vi "Bind Terminal Enabled State.vi"(4 "FALSE State (Disabled and Grayed Out)":T1(ring), 6 "TRUE State (Enabled)":T1(ring), 7 "Initial State (T)":bool=TRUE, 8 "error in (no error)":errorcluster, 9 "Datum Name (\"\"=Use Control Label)":string, 10 "Ctl Refnum":refnum<vi>, 11 "IViewable in":refnum<class "IViewable.lvclass">) -> (0 "error out":errorcluster, 3 "IViewable out":refnum<class "IViewable.lvclass">)   [LabVIEW 2015, in "IViewable.lvlib" / "IViewable.lvclass"]
doc: "Bind the enabled state of a control terminal (control or indicator) to a published Boolean or Numeric datum. Specify the logical relationship between datum vale and terminal state by wiring the optional input terminals.\n\nDefault for Boolean:\nPublished TRUE = Enabled\nPublished FALSE = Disabled and Grayed Out\n\nDefault for Numeric:\nPublised value greater than 0 = Enabled\nPublished value NOT greater than 0 = Disabled and Grayed Out"
uses:
  IViewable.lvclass
  <vilib>/ActorFramework/Actor/Actor.lvclass/Actor.ctl
  <vilib>/ActorFramework/Message Enqueuer/Message Enqueuer.lvclass/Message Enqueuer.ctl
  SubscriptionPolicy/ValueChangeSubscription/ValueChangeSubscription.lvclass/ValueChangeSubscription.ctl
  IMediator/SubscriptionRequest/SubscriptionRequest.lvclass/SubscriptionRequest.ctl
  IObserver/IObserver Messages/Subscribe Msg/Subscribe Msg.lvclass/Subscribe Msg.ctl
  <vilib>/ActorFramework/Message Enqueuer/Init from Existing Queue.vi
  <vilib>/ActorFramework/Message Enqueuer/Enqueue.vi
  <vilib>/ActorFramework/Message Priority Queue/Priority Enqueue.vi
  SubscriptionPolicy/ValueChangeSubscription/ValueChangeSubscription.lvclass
  <vilib>/ActorFramework/Message Enqueuer/Message Enqueuer.lvclass
  IMediator/SubscriptionRequest/SubscriptionRequest.lvclass
  IObserver/IObserver Messages/Subscribe Msg/Subscribe Msg.lvclass
  <vilib>/ActorFramework/Actor/Actor.lvclass
  IMediator/ISubscriptionPolicy/ISubscriptionPolicy.lvclass
  Transport/TerminalEnabledStateBinding/TerminalEnabledStateBinding.lvclass
  <vilib>/Utility/Data Type/NI_Data Type.lvlib
panel:
  in  "Datum Type (Boolean)":variant
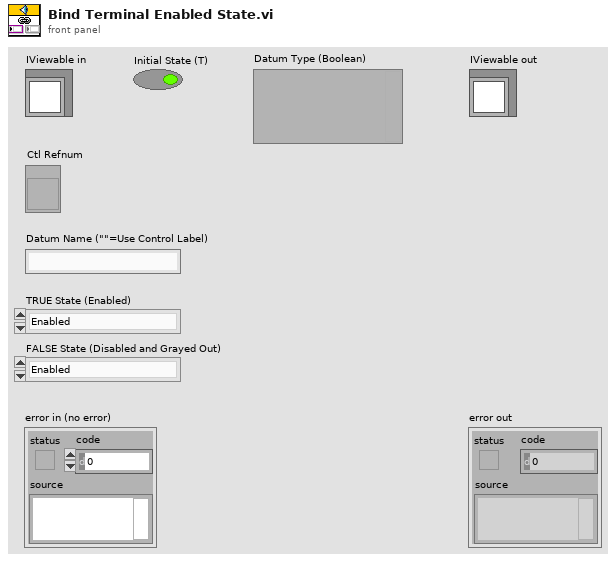
[diagram p1: front panel]
types:
  T1 = enum8{"Enabled", "Disabled", "Disabled and Grayed Out"}
  T2 = typedef "NI_Data Type.lvlib/Data Type.ctl" = enum8{"Invalid Type", "Void", "I8", "I16", "I32", "I64", "U8", "U16", "U32", "U64", "Single Float", "Double Float", "Extended Float", "Single Complex", "Double Complex", "Extended Complex", "Enum U8", "Enum U16", "Enum U32", "Enum U64", "Single Float With Unit", "Double Float With Unit", "Extended Float With Unit", "Single Complex with Unit", "Double Complex with Unit", "Extended Complex with Unit", "Boolean", "String", "Path", "Picture", "Tag", "Array", "Cluster", "Variant", "LV Variant", "Waveform", "Timestamp", "Digital Waveform", "Digital Data", "ExpressData", "Refnum", "External Data", "VI", "Poly VI", "LabVIEW Class Instance", "Fixed Point"}
  T3 = typedef "IMediator.lvlib/ISubscriptionPolicy.lvclass/ISubscriptionPolicy Reference.ctl" = refnum<data-value>
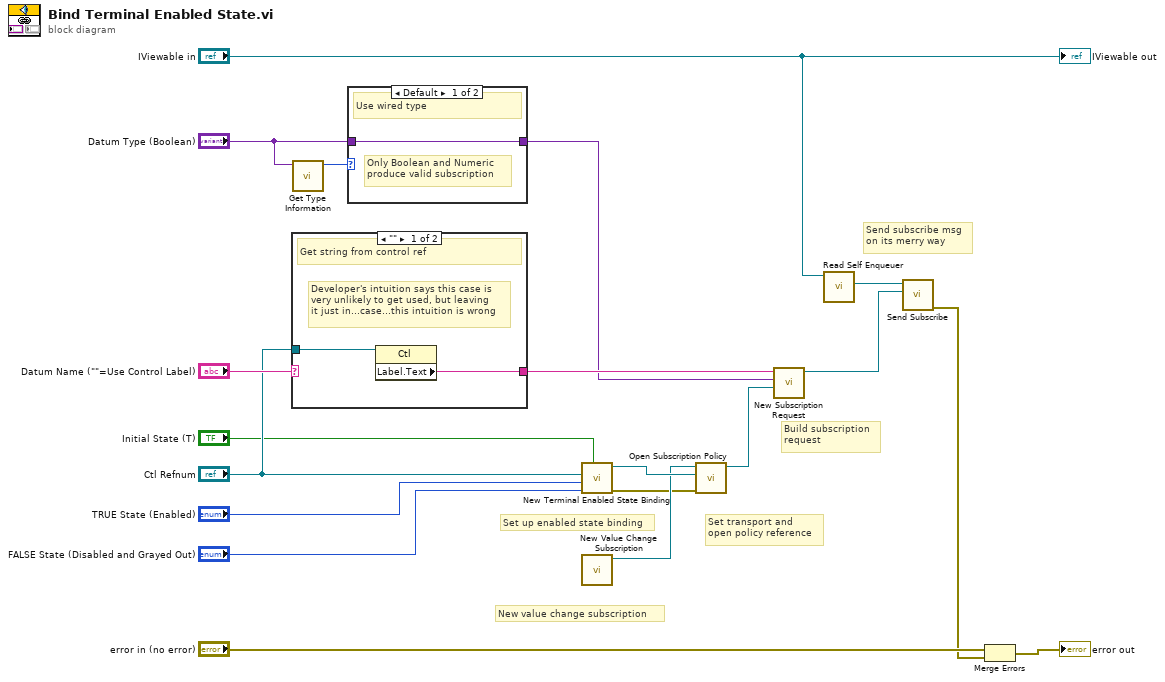
[diagram p0: block diagram]
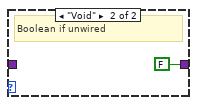
[diagram p2: hidden frame]
diagram:
  # "New value change subscription"
  # "Set transport and\nopen policy reference"
  # "Send subscribe msg\non its merry way"
  # "Build subscription\nrequest"
  # "Set up enabled state binding"
  n1 = case shown="\"\"" "Datum Name (\"\"=Use Control Label)" {
    selector: "Datum Name (\"\"=Use Control Label)" -> [_ w22]
    tunnel: [w20 w22] -> w12
    tunnel: "Ctl Refnum" -> [w21 _]
    frame "" {
      # "Developer's intuition says this case is\nvery unlikely to get used, but leaving\nit just in...case...this intuition is wrong"
      # "Get string from control ref"
      n2 = property class="Ctl"(reference=w21) -> ("Label.Text"=w20:string)  [unwired: 1 in, 2 out]
    }
    frame Default {
      # "Use string wired to input terminal"
    }
  }
  n3 = call <vilib>:"Get Type Information.vi"("Variant"="Datum Type (Boolean)") -> ("Type"=w4:T2)  [unwired: 6 in, 4 out]
  n4 = case shown="Default" w4 {
    tunnel: [w23 FALSE] -> w3
    tunnel: "Datum Type (Boolean)" -> [w23 _]
    frame Default {
      # "Only Boolean and Numeric\nproduce valid subscription"
      # "Use wired type"
    }
    frame "Void" {
      # "Boolean if unwired"
    }
  }
  n5 = call "New Terminal Enabled State Binding.vi"("Initial State (T)"="Initial State (T)", "FALSE State (Disabled and Grayed Out)"="FALSE State (Disabled and Grayed Out)", "TRUE State (Enabled)"="TRUE State (Enabled)", "Control"="Ctl Refnum") -> ("error out"=w5:errorcluster, "TerminalEnabledStateBinding Out"=w10:refnum<class "TerminalEnabledStateBinding.lvclass">)  [unwired: 6 in]
  n6 = call "New Value Change Subscription.vi"() -> ("ValueChangeSubscription Out"=w9:refnum<class "ValueChangeSubscription.lvclass">)  [unwired: 11 in]
  n7 = call "Open Subscription Policy.vi"("error in (no error)"=w5, "Transport"=w10, "SubscriptionPolicy"=w9) -> ("Subscription Policy"=w1:T3)  [unwired: 7 in, 1 out]
  n8 = call "New Subscription Request.vi"("Subscription Policy"=w1, "Type"=w3, "Datum Name"=w12) -> ("SubscriptionRequest"=w16:refnum<class "SubscriptionRequest.lvclass">)  [unwired: 8 in]
  n9 = call <vilib>:"Read Self Enqueuer.vi"("Actor"="IViewable in") -> ("Self Enqueuer"=w17:refnum<class "Message Enqueuer.lvclass">)  [unwired: 10 in]
  n10 = call "Send Subscribe.vi"("SubscriptionRequest"=w16, "Message Enqueuer"=w17) -> ("error out"=w14:errorcluster)  [unwired: 8 in, 1 out]
  n11 = Merge Errors("error in (no error)", w14) -> (→"error out":errorcluster)
  "IViewable out" <- "IViewable in"
